vi "GPR Facade.vi"(0 "Data In":T11, 2 "Display State In":T2, 3 "Container State":T10) -> (6 "Data Out":T11, 7 "Display State Out":T2, 8 "Action":T1)   [LabVIEW 2009, in "GPR.xctl"]
uses:
  GPR.xctl
  GPR Data.ctl
  <vilib>/_xctls/Container State.ctl
  GPR State.ctl
  Controls/GPR Graph Info.ctl
  Controls/Display Types.ctl
  Controls/Display Info.ctl
  Controls/Trace Options.ctl
  Controls/Fill Options.ctl
  Controls/Intensity Options.ctl
  Controls/Color Scales.ctl
  <vilib>/_xctls/Action.ctl
  <vilib>/_xctls/XControlSupport.lvlib
panel:
  out "Picture":picture
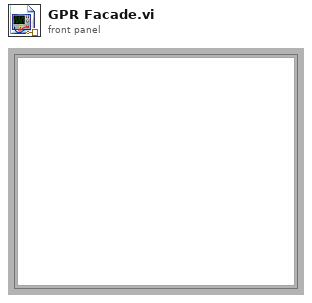
[diagram p1: front panel]
types:
  T1 = typedef "XControlSupport.lvlib/Action.ctl" = cluster{"Data Changed?":bool, "State Changed?":bool, "Action Name":string}
  T2 = typedef "GPR.xctl/GPR State.ctl" = cluster{"GPR Graph Info":T3, "Transpose Data":bool, "Run-time Edit":bool, "Clear Request":bool}
  T3 = typedef "GPR Graph Info.ctl" = cluster{"Display Type":T4, "Display Info":T5, "Trace Options":T6, "Intensity Options":T8}
  T4 = typedef "Display Types.ctl" = enum16{"Intensity Plot", "Wiggle Trace"}
  T5 = typedef "Display Info.ctl" = cluster{"X Scale":cluster{"X Scale Label":bool, "X Scale Name":string, "X Scale Visible":bool, "dx":dbl}, "Y Scale":cluster{"X Scale Label":bool, "X Scale Name":string, "X Scale Visible":bool, "dt":dbl}, "BackGround Color":u32}
  T6 = typedef "Trace Options.ctl" = cluster{"Trace Amplitude":dbl, "Trace Color":u32, "Fill options":T7}
  T7 = typedef "Fill Options.ctl" = enum32{"No Fill", "Fill Positive", "Fill Negative"}
  T8 = typedef "Intensity Options.ctl" = cluster{"Color Scale":T9}
  T9 = typedef "Color Scales.ctl" = enum16{"RGB", "RWB", "BGR", "BWR", "BW", "WB"}
  T10 = typedef "XControlSupport.lvlib/Container State.ctl" = cluster{"Indicator?":bool, "Run Mode?":bool, " Refnum":refnum<vi>}
  T11 = typedef "GPR.xctl/GPR Data.ctl" = dbl[][]
  T12 = typedef "LVBoundsTypeDef.ctl" = cluster{"Width":u32, "Height":u32}
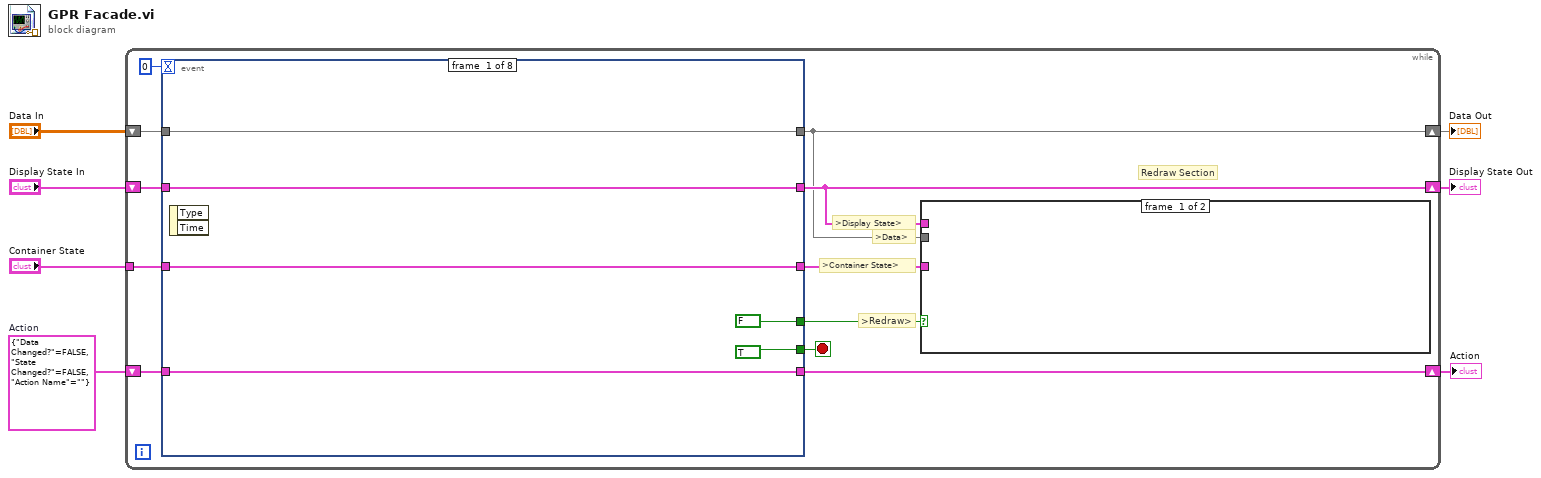
[diagram p0: block diagram]
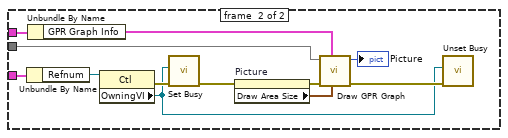
[diagram p2: hidden frame]
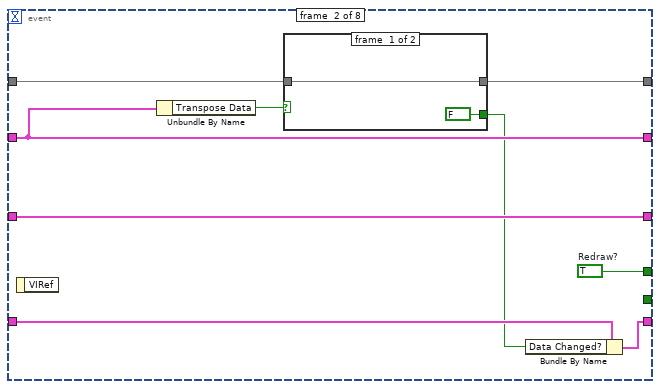
[diagram p3: hidden frame]
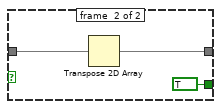
[diagram p4: hidden frame]
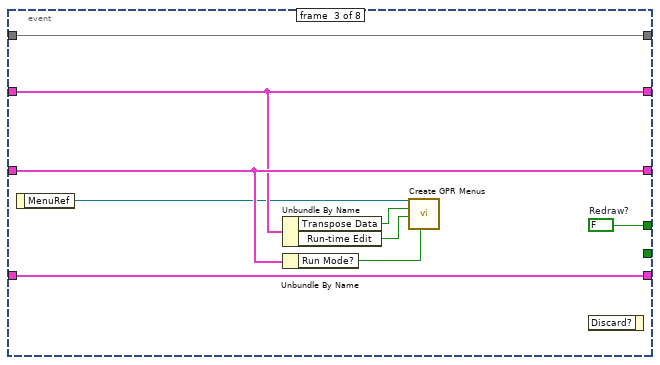
[diagram p5: hidden frame]
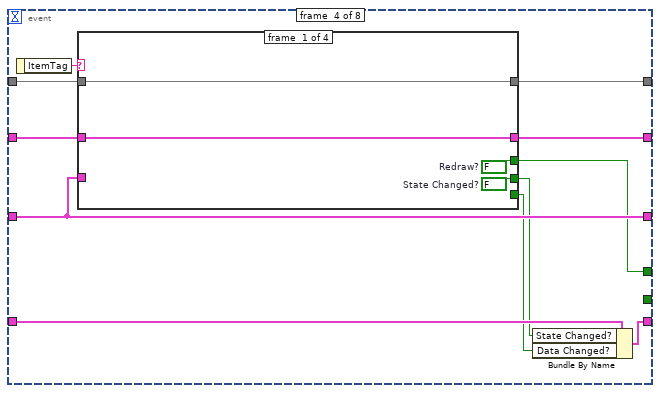
[diagram p6: hidden frame]
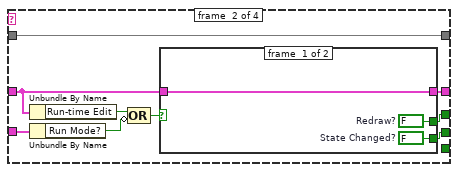
[diagram p7: hidden frame]
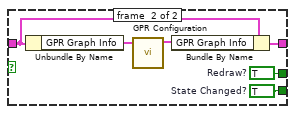
[diagram p8: hidden frame]
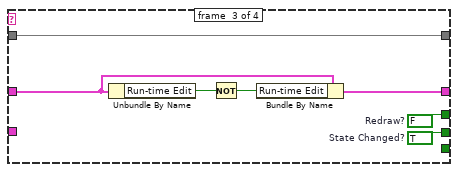
[diagram p9: hidden frame]
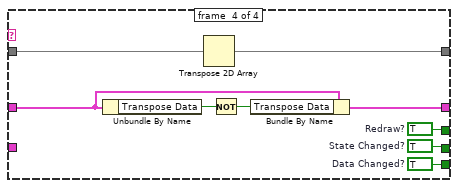
[diagram p10: hidden frame]
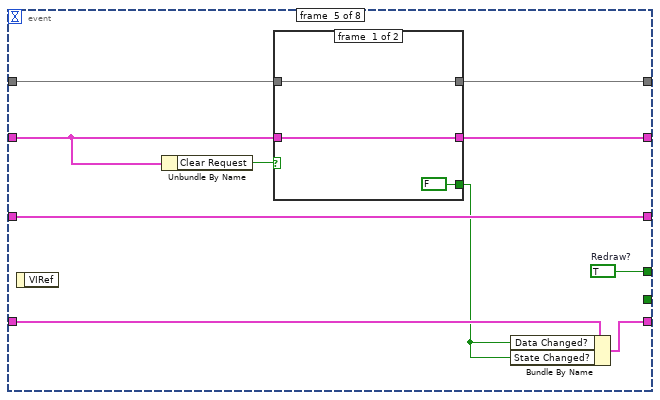
[diagram p11: hidden frame]
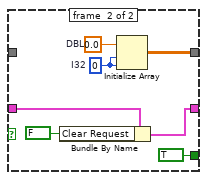
[diagram p12: hidden frame]
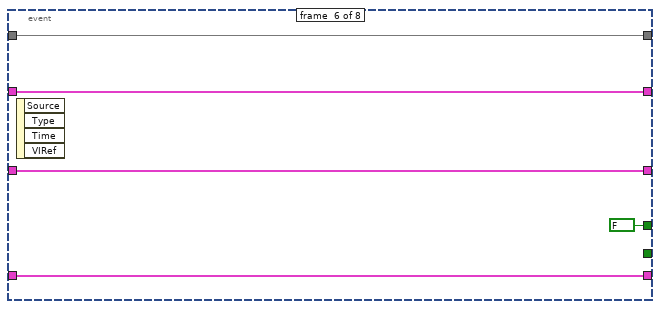
[diagram p13: hidden frame]
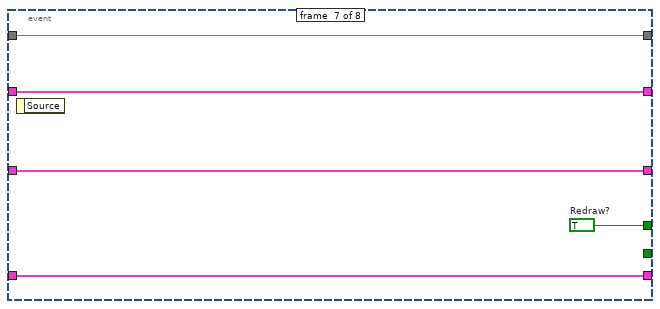
[diagram p14: hidden frame]
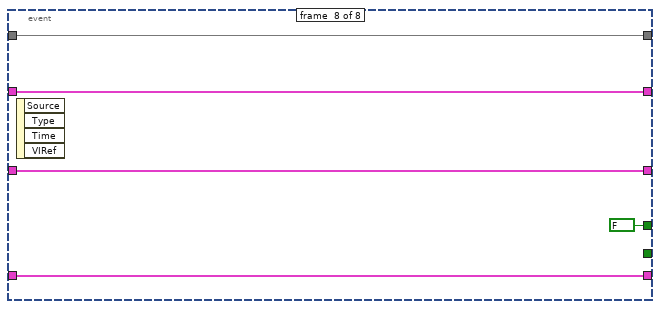
[diagram p15: hidden frame]
diagram:
  w1 = T1 {"Data Changed?"=FALSE, "State Changed?"=FALSE, "Action Name"=""}  # Action
  n1 = while {
    shift-right: [w9] -> w4
    shift-left: "Display State In" -> [w18]
    tunnel: "Container State" -> [w15]
    shift-right: [w8] -> w7
    shift-left: "Data In" -> [w14]
    shift-right: [w12] -> w2
    shift-left: w1 -> [w13]
    stop <- w17 stop-if-true
    # "Redraw Section"
    # ">Redraw>"
    # ">Container State>"
    # ">Data>"
    # ">Display State>"
    n2 = event shown="[3] \"Picture\": Shortcut Menu Selection (User)" {
      selector: _ -> [_ _ _ _ _ _ _ _]
      dyn-events: _ -> [_ _ _ _ _ _ _ _]
      timeout: 0 -> [_ _ _ _ _ _ _ _]
      tunnel: w18 -> [w34 w42 w56 w67 w113 w133 w137 w143]
      tunnel: [w34 w42 w56 w70 w111 w133 w137 w143] -> w9
      tunnel: [TRUE _ _ _ _ _ _ _] -> w17
      tunnel: w15 -> [w31 w45 w57 w65 w117 w129 w136 w140]
      tunnel: w14 -> [w33 w43 w55 w64 w112 w132 w138 w142]
      tunnel: [w33 w40 w55 w63 w110 w132 w138 w142] -> w8
      tunnel: [w35 w38 w58 w68 w115 w131 w134 w141] -> w12
      tunnel: w13 -> [w35 w39 w58 w69 w116 w131 w134 w141]
      tunnel: [FALSE ("Redraw?") w44 w59 w62 w118 FALSE ("Redraw?") w135 FALSE ("Redraw?")] -> w11
      tunnel: [w31 w45 w57 w65 w117 w129 w136 w140] -> w10
      event #0 {
        n3 = event-data() -> ()  [unwired: 1 in, 2 out]
      }
      event #1 {
        w44 = TRUE  # Redraw?
        n4 = event-data() -> ()  [unwired: 1 in, 1 out]
        n5 = Unbundle By Name(w42) -> ("Transpose Data"=w41:bool)
        n6 = case shown="True" w41 {
          tunnel: w43 -> [w47 w50]
          tunnel: [w47 w49] -> w40
          tunnel: [FALSE ("Data Changed?") TRUE ("Data Changed?")] -> w37
          frame #0 {
          }
          frame #1 {
            n7 = Transpose 2D Array(2D array=w50) -> (transposed array=w49:T11)
          }
        }
        n8 = Bundle By Name(cluster=w39, "Data Changed?"=w37) -> (w38:T1)
      }
      event #2 {
        w59 = FALSE  # Redraw?
        n9 = event-data() -> ("MenuRef"=w54:refnum<k9>)  [unwired: 1 in]
        n10 = Unbundle By Name(w56) -> ("Transpose Data"=w53:bool, "Run-time Edit"=w52:bool)
        n11 = Unbundle By Name(w57) -> ("Run Mode?"=w51:bool)
        n12 = call "Create GPR Menus.vi"("Run Mode"=w51, "Run-time Edit"=w52, "Transpose data"=w53, "menu reference"=w54) -> ()  [unwired: 6 in, 2 out]
        n13 = event-data() -> ()  [unwired: 2 in, 1 out]
      }
      event #3 {
        n14 = event-data() -> ("ItemTag"=w66:string)  [unwired: 1 in]
        n15 = case shown="\"GPR_PROPERTIES\"" w66 {
          tunnel: w67 -> [w73 w77 w95 w105]
          tunnel: [w73 w83 w94 w104] -> w70
          tunnel: [w72 w79 w97 w107] -> w62
          tunnel: w65 -> [_ w78 _ _]
          tunnel: w64 -> [w74 w76 w99 w102]
          tunnel: [w74 w76 w99 w101] -> w63
          tunnel: [w71 w75 w98 w108] -> w61
          tunnel: [_ _ _ w100] -> w60
          frame #0 {
            w71 = FALSE  # State Changed?
            w72 = FALSE  # Redraw?
          }
          frame #1 {
            n16 = Unbundle By Name(w77) -> ("Run-time Edit"=w81:bool)
            n17 = Unbundle By Name(w78) -> ("Run Mode?"=w82:bool)
            n18 = Compound Arithmetic op=OR(w81, invert w82) -> (w80:bool)
            n19 = case shown="False" w80 {
              tunnel: w77 -> [w86 w91]
              tunnel: [w86 w89] -> w83
              tunnel: [w85 w88] -> w79
              tunnel: [w84 w87] -> w75
              frame #0 {
                w84 = FALSE  # State Changed?
                w85 = FALSE  # Redraw?
              }
              frame #1 {
                w87 = TRUE  # State Changed?
                w88 = TRUE  # Redraw?
                n20 = Unbundle By Name(w91) -> ("GPR Graph Info"=w92:T3)
                n21 = call "GPR Configuration.vi"("GPR Graph Info In"=w92) -> ("GPR Graph Info Out"=w90:T3)  [unwired: 9 in, 1 out]
                n22 = Bundle By Name(cluster=w91, "GPR Graph Info"=w90) -> (w89:T2)
              }
            }
          }
          frame #2 {
            w97 = FALSE  # Redraw?
            w98 = TRUE  # State Changed?
            n23 = Unbundle By Name(w95) -> ("Run-time Edit"=w96:bool)
            n24 = Not(x=w96) -> (.not. x?=w93:bool)
            n25 = Bundle By Name(cluster=w95, "Run-time Edit"=w93) -> (w94:T2)
          }
          frame #3 {
            w100 = TRUE  # Data Changed?
            w107 = TRUE  # Redraw?
            w108 = TRUE  # State Changed?
            n26 = Unbundle By Name(w105) -> ("Transpose Data"=w106:bool)
            n27 = Transpose 2D Array(2D array=w102) -> (transposed array=w101:T11)
            n28 = Not(x=w106) -> (.not. x?=w103:bool)
            n29 = Bundle By Name(cluster=w105, "Transpose Data"=w103) -> (w104:T2)
          }
        }
        n30 = Bundle By Name(cluster=w69, "State Changed?"=w61, "Data Changed?"=w60) -> (w68:T1)
      }
      event #4 {
        w118 = TRUE  # Redraw?
        n31 = event-data() -> ()  [unwired: 1 in, 1 out]
        n32 = Unbundle By Name(w113) -> ("Clear Request"=w114:bool)
        n33 = case shown="False" w114 {
          tunnel: w113 -> [w121 w128]
          tunnel: w112 -> [w120 _]
          tunnel: [w121 w124] -> w111
          tunnel: [w120 w127] -> w110
          tunnel: [FALSE ("Clear Request") TRUE ("Clear Request")] -> w109
          frame #0 {
          }
          frame #1 {
            w125 = 0  # I32
            w126 = 0.0  # DBL
            n34 = Bundle By Name(cluster=w128, "Clear Request"=FALSE) -> (w124:T2)
            n35 = Initialize Array "Initialize Array"(w126, w125, w125) -> (w127:dbl[][])
          }
        }
        n36 = Bundle By Name(cluster=w116, "Data Changed?"=w109, "State Changed?"=w109) -> (w115:T1)
      }
      event #5 {
        n37 = event-data() -> ()  [unwired: 1 in, 4 out]
      }
      event #6 {
        w135 = TRUE  # Redraw?
        n38 = event-data() -> ()  [unwired: 1 in, 1 out]
      }
      event #7 {
        n39 = event-data() -> ()  [unwired: 1 in, 4 out]
      }
    }
    n40 = case shown="True" w11 {
      tunnel: w10 -> [_ w30]
      tunnel: w9 -> [_ w26]
      tunnel: w8 -> [_ w24]
      frame #0 {
      }
      frame #1 {
        n41 = Unbundle By Name(w30) -> ("Refnum"=w29:refnum<vi>)
        n42 = Unbundle By Name(w26) -> ("GPR Graph Info"=w25:T3)
        n43 = property on="Property Node" class="Ctl"(reference=w29) -> (error out=w28:errorcluster, "OwningVI"=w19:refnum<vi>)  [unwired: 1 in, 1 out]
        n44 = call <vilib>:"Set Busy.vi"("error in (no error)"=w28, "VI reference (current VI)"=w19) -> ("error out"=w27:errorcluster)  [unwired: 8 in, 1 out]
        n45 = property on="Picture" class="Pict"(error in=w27) -> (error out=w23:errorcluster, "Draw Area Size"=w21:T12)  [unwired: 1 in, 1 out]
        n46 = call "Draw GPR Graph.vi"("Draw Area Size"=w21, "Graph Info"=w25, "error in"=w23, "Data"=w24) -> ("error out"=w20:errorcluster, "picture out"=→"Picture":picture)  [unwired: 6 in]
        n47 = call <vilib>:"Unset Busy.vi"("error in (no error)"=w20, "VI reference (current VI)"=w19) -> ()  [unwired: 9 in, 1 out]
      }
    }
  }
  "Display State Out" <- w4
  "Data Out" <- w7
  "Action" <- w2
